vi "Set Waveform Display Intensity.vi"(8 "error in (no error)":errorcluster, 10 "Intensity (1-100)":i8=1 min=1 max=100 step=1, 11 "MSOX6004 in":refnum<class "MSOX6004.lvclass">) -> (0 "error out":errorcluster, 3 "MSOX6004 out":refnum<class "MSOX6004.lvclass">)   [LabVIEW 2018, in "MSOX6004.lvlib" / "MSOX6004.lvclass"]
doc: "This Override is used to change the display intensity level for the oscilloscope waveforms."
uses:
  MSOX6004.lvclass
  MSOX6004.lvclass/MSOX6004.ctl
  <instrlib>/Keysight InfiniiVision/Keysight InfiniiVision.lvlib
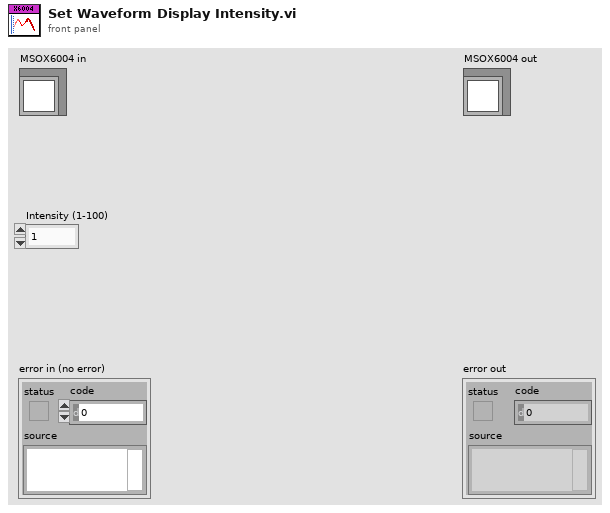
[diagram p1: front panel]
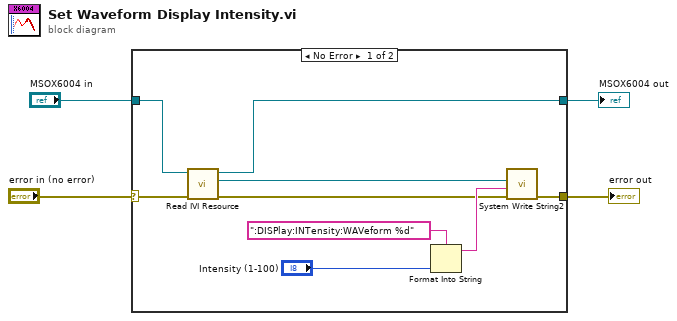
[diagram p0: block diagram]
diagram:
  n1 = case shown="No Error" "error in (no error)" {
    selector: "error in (no error)" -> [w12 w15]
    tunnel: [w5 w15] -> w3
    tunnel: [w11 w14] -> w2
    tunnel: "MSOX6004 in" -> [w13 w14]
    frame No Error {
      n2 = call "Read IVI Resource.vi"("error in (no error)"=w12, "MSOX6004 in"=w13) -> ("error out"=w8:errorcluster, "IVI Resource"=w7:refnum<k15>, "MSOX6004 out"=w11:refnum<class "MSOX6004.lvclass">)  [unwired: 7 in]
      n3 = Format Into String(format string=":DISPlay:INTensity:WAVeform %d", "Intensity (1-100)") -> (resulting string=w9:string)  [unwired: 2 in, 1 out]
      n4 = call <instrlib>:"System Write String2.vi"("error in (no error)"=w8, "Data"=w9, "instrument handle"=w7) -> ("error out"=w5:errorcluster)  [unwired: 7 in, 1 out]
    }
    frame Error {
    }
  }
  "error out" <- w3
  "MSOX6004 out" <- w2
